vi "FunctionalGlobals.vi"(0 "FG_Control":enum16{"Initialize", "PowerRead", "PowerWrite"}(ring), 5 "FG_IN":cluster{"PowerIn":dbl} {"PowerIn" format="%.2p"}) -> (6 "FG_OUT":cluster{"PowerOut":dbl} {"PowerOut" format="%.2p"})   [LabVIEW 2012]
panel:
  out "PowerOut":dbl format="%.2p"
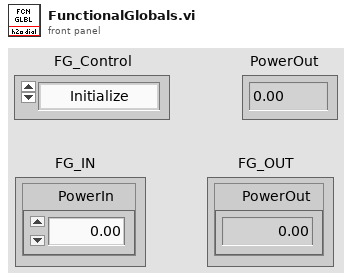
[diagram p1: front panel]
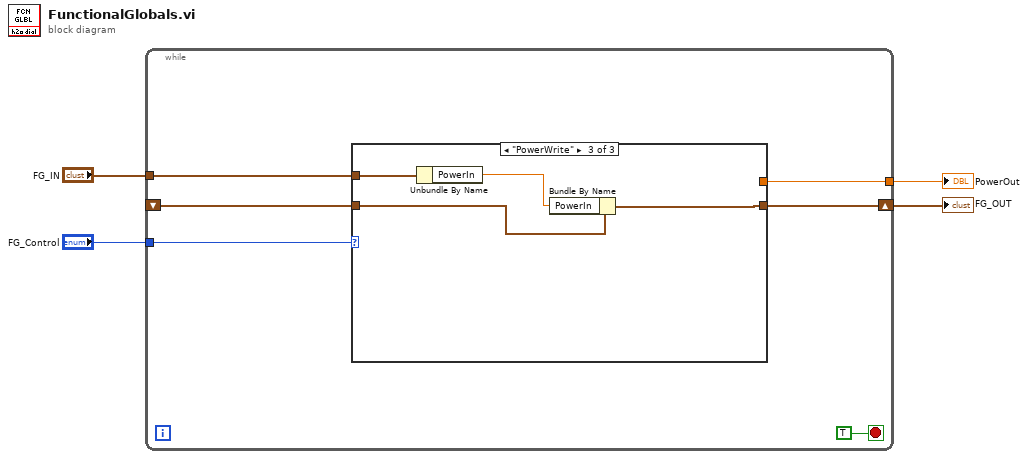
[diagram p0: block diagram]
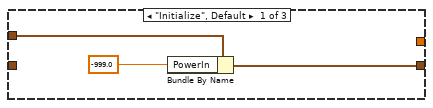
[diagram p2: hidden frame]
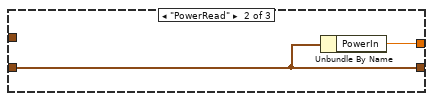
[diagram p3: hidden frame]
diagram:
  n1 = while {
    shift-right: [w9] -> w2
    shift-left: _ -> [w8]
    tunnel: "FG_Control" -> [w10]
    tunnel: "FG_IN" -> [w6]
    tunnel: [w5] -> w1
    stop <- TRUE stop-if-true
    n2 = case shown="\"PowerWrite\"" w10 {
      tunnel: [w11 w15 w19] -> w9
      tunnel: w8 -> [_ w15 w18]
      tunnel: w6 -> [w13 _ w17]
      tunnel: [_ w14 _] -> w5
      frame "Initialize", Default {
        n3 = Bundle By Name(cluster=w13, "PowerIn"=-999.0) -> (w11:cluster{"PowerIn":dbl})
      }
      frame "PowerRead" {
        n4 = Unbundle By Name(w15) -> ("PowerIn"=w14:dbl)
      }
      frame "PowerWrite" {
        n5 = Unbundle By Name(w17) -> ("PowerIn"=w16:dbl)
        n6 = Bundle By Name(cluster=w18, "PowerIn"=w16) -> (w19:cluster{"PowerIn":dbl})
      }
    }
  }
  "FG_OUT" <- w2
  "PowerOut" <- w1
